vi "Get Data Word Format.vi"(8 "error in":errorcluster, 11 "logging ref":T2=18446744073709551615 format="%.0x") -> (0 "error out":errorcluster, 2 "data word format":T1, 3 "logging ref out":T2 format="%.0x")   [LabVIEW 2024, in "AIM ARINC 429 Scripting.lvlib"]
doc: "Returns the format of data words in the log file."
uses:
  AIM ARINC 429 Scripting.lvlib
  <vilib>/NI VeriStand/Custom Device API/Custom Device Item Ref.ctl
  Shared/Data Word Format.ctl
  Constants.vi
  <vilib>/NI VeriStand/Custom Device API/Get Item Property (String).vi
  <vilib>/NI VeriStand/Custom Device API/Custom Device API.lvlib
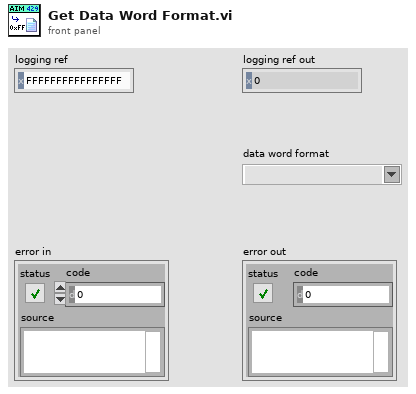
[diagram p1: front panel]
types:
  T1 = typedef "Data Word Format.ctl" = string
  T2 = typedef "Custom Device API.lvlib/Custom Device Item Ref.ctl" = u64
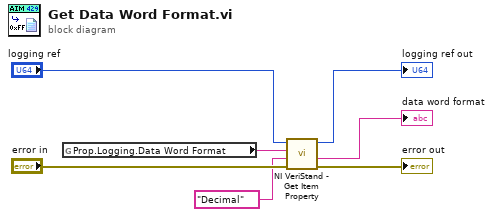
[diagram p0: block diagram]
diagram:
  n1 = global read "Constants.vi" "Prop.Logging.Data Word Format"() -> (w7:string)
  n2 = call-poly <vilib>:"NI VeriStand - Get Item Property.vi"("error in (no error)"="error in", "Default Value"=T1 "Decimal" ("data word format"), "Property Name"=w7, "Item Ref in"="logging ref") -> ("error out"=→"error out":errorcluster, "Value"=→"data word format":string, "Item Ref out"=→"logging ref out":T2)  [unwired: 4 in, 1 out]
